vi "AutoDrive.vi"(10 "Target":dbl, 11 "Drive Effort":dbl) -> ()   [LabVIEW 2017]
uses:
  2017_Steamworks/Programming_Team/Competition/Worlds/Labview/Global 2.vi
  <vilib>/Rock Robotics/WPI/ThirdParty/Phoenix-LabVIEW/Motor Controller/Controls/CTRE_Phoenix_MotorControl_ControlMode.ctl
panel:
  in  "Scaling Factor":dbl
  in  "kD":dbl
  in  "kP":dbl
  in  "Scaling Factor":dbl=16.0 format="%#_13g"
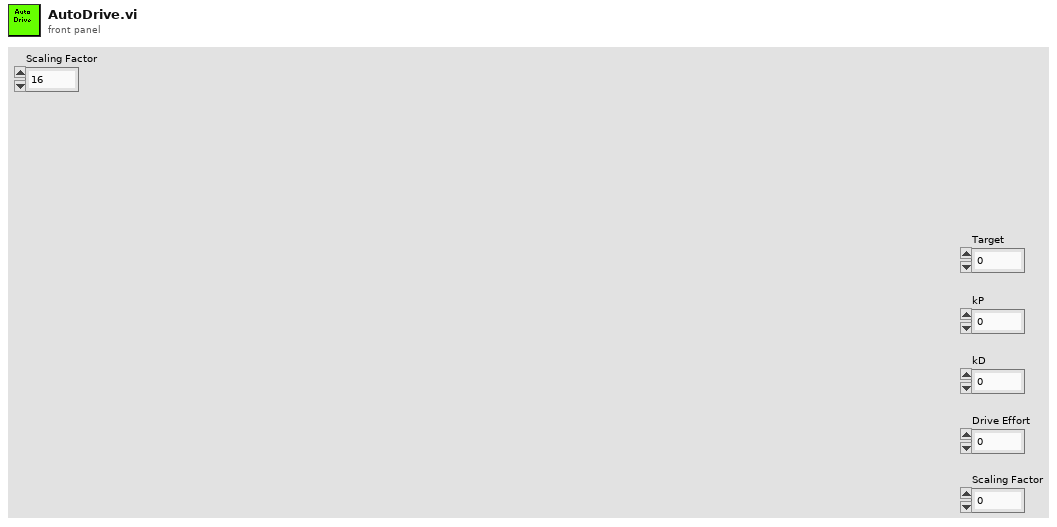
[diagram p1: front panel]
types:
  T1 = typedef "CTRE_Phoenix_MotorControl_ControlMode.ctl" = u16
  T2 = typedef "WPI_MotorControlDeviceRef.ctl" = cluster{"DeviceStatus":errorcluster, "Type":T3, "PWM":cluster{"PWM Channel":T4, "DeadBand":T5}, "CAN":cluster{"Device Number":u8, "SetOutput VI Ref":variant, "GetOutput VI Ref":variant, "Enable VI Ref":variant, "Disable VI Ref":variant, "Data":variant}, "Invert":bool, "DIO PWM":cluster{"PWM \"Enable\" Channel":T4, "DIOChannel":T6, "PWM Rate":dbl}}
  T3 = typedef "WPI_MotorControlType.ctl" = enum16{"PWM", "CAN", "DIO PWM"}
  T4 = typedef "FPGA_DIOPWMChannel.ctl" = enum8{"PWM 0", "PWM 1", "PWM 2", "PWM 3", "PWM 4", "PWM 5", "PWM 6", "PWM 7", "PWM 8", "PWM 9", "PWM MXP 0", "PWM MXP 1", "PWM MXP 2", "PWM MXP 3", "PWM MXP 4", "PWM MXP 5", "PWM MXP 6", "PWM MXP 7", "PWM MXP 8", "PWM MXP 9", "Invalid"}
  T5 = typedef "WPI_PWMDeadband.ctl" = cluster{"Name":string, "maxPositivePwm":i32, "minPositivePwm":i32, "centerPwm":i32, "maxNegativePwm":i32, "minNegativePwm":i32, "angularRange":u16}
  T6 = typedef "FPGA_DIOChannel.ctl" = enum8{"DIO 0", "DIO 1", "DIO 2", "DIO 3", "DIO 4", "DIO 5", "DIO 6", "DIO 7", "DIO 8", "DIO 9", "DIO MXP 0", "DIO MXP 1", "DIO MXP 2", "DIO MXP 3", "DIO MXP 4", "DIO MXP 5", "DIO MXP 6", "DIO MXP 7", "DIO MXP 8", "DIO MXP 9", "DIO MXP 10", "DIO MXP 11", "DIO MXP 12", "DIO MXP 13", "DIO MXP 14", "DIO MXP 15", "SPI Port CS1", "SPI Port CS2", "SPI Port CS3", "SPI Port MISO", "SPI Port MOSI", "Invalid"}
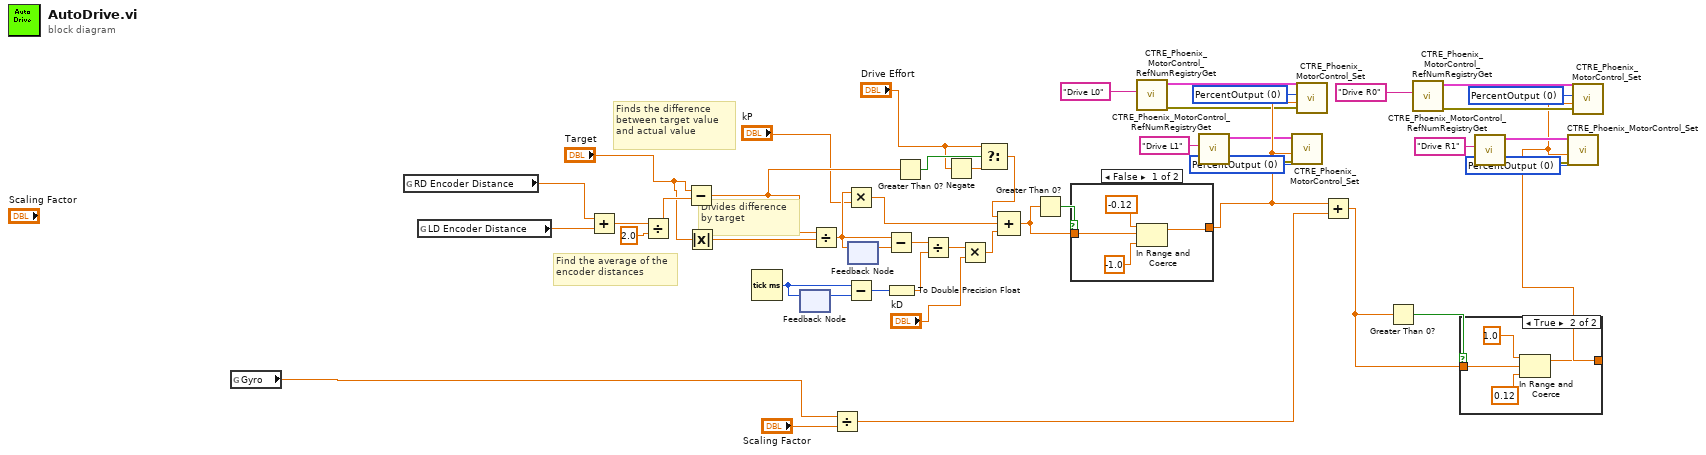
[diagram p0: block diagram]
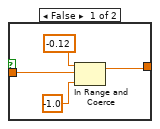
[diagram p2: hidden frame]
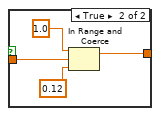
[diagram p3: hidden frame]
diagram:
  w1 = T1 0 items=["PercentOutput"=0, "Position"=1, "Velocity"=2, "Current"=3, "Follower"=5, "MotionProfile"=6, "MotionMagic"=7, "MotionMagicArc"=8, "MotionProfileArc"=10, "Disabled"=15] ("Control Mode")
  w2 = T1 0 items=["PercentOutput"=0, "Position"=1, "Velocity"=2, "Current"=3, "Follower"=5, "MotionProfile"=6, "MotionMagic"=7, "MotionMagicArc"=8, "MotionProfileArc"=10, "Disabled"=15] ("Control Mode")
  w3 = T1 0 items=["PercentOutput"=0, "Position"=1, "Velocity"=2, "Current"=3, "Follower"=5, "MotionProfile"=6, "MotionMagic"=7, "MotionMagicArc"=8, "MotionProfileArc"=10, "Disabled"=15] ("Control Mode")
  w4 = T1 0 items=["PercentOutput"=0, "Position"=1, "Velocity"=2, "Current"=3, "Follower"=5, "MotionProfile"=6, "MotionMagic"=7, "MotionMagicArc"=8, "MotionProfileArc"=10, "Disabled"=15] ("Control Mode")
  # "Divides difference by target"
  # "Finds the difference between target value and actual value"
  # "Find the average of the encoder distances"
  n1 = global read "Global 2.vi" "Gyro"() -> (w46:dbl)
  n2 = global read "Global 2.vi" "RD Encoder Distance"() -> (w30:dbl)
  n3 = global read "Global 2.vi" "LD Encoder Distance"() -> (w31:dbl)
  n4 = Add(x=w30, y=w31) -> (x+y=w45:dbl)
  n5 = Divide(x=w45, y=2.0) -> (x/y=w43:dbl)
  n6 = Subtract(x="Target", y=w43) -> (x-y=w25:dbl)
  n7 = Absolute Value(x="Target") -> (abs(x)=w27:dbl)
  n8 = Tick Count (ms)() -> (millisecond timer value=w40:u32)
  n9 = feedback #1() -> (w41:u32)  [unwired: 1 in]
  n10 = feedback-in #1(w40) -> ()
  n11 = Divide(x=w25, y=w27) -> (x/y=w26:dbl)
  n12 = Divide(x=w46, y="Scaling Factor") -> (x/y=w47:dbl)
  n13 = Multiply(x=w26, y="kP") -> (x*y=w35:dbl)
  n14 = Subtract(x=w40, y=w41) -> (x-y=w38:u32)
  n15 = feedback #2() -> (w42:dbl)  [unwired: 1 in]
  n16 = feedback-in #2(w26) -> ()
  n17 = Subtract(x=w26, y=w42) -> (x-y=w39:dbl)
  n18 = To Double Precision Float(number=w38) -> (double precision float=w37:dbl)
  n19 = Greater Than 0?(x=w25) -> (x > 0?=w24:bool)
  n20 = Divide(x=w39, y=w37) -> (x/y=w36:dbl)
  n21 = Negate(x="Drive Effort") -> (-x=w23:dbl)
  n22 = Multiply(x=w36, y="kD") -> (x*y=w34:dbl)
  n23 = Select(t="Drive Effort", s=w24, f=w23) -> (s? t:f=w22:dbl)
  n24 = Compound Arithmetic op=ADD(w22, w35, w34) -> (w32:dbl)
  n25 = Greater Than 0?(x=w32) -> (x > 0?=w33:bool)
  n26 = case shown="False" w33 {
    tunnel: [w50 w55] -> w17
    tunnel: w32 -> [w51 w54]
    frame False {
      n27 = In Range and Coerce(upper limit=-0.12, x=w51, lower limit=-1.0) -> (coerced(x)=w50:dbl)  [unwired: 1 out]
    }
    frame True {
      n28 = In Range and Coerce(upper limit=1.0, x=w54, lower limit=0.12) -> (coerced(x)=w55:dbl)  [unwired: 1 out]
    }
  }
  n29 = call <vilib>:"CTRE_Phoenix_MotorControl_RefNumRegistryGet.vi"("refnum name"="Drive L0") -> ("error out"=w12:errorcluster, "PhoenixMotorControlDevRef"=w13:T2)  [unwired: 9 in]
  n30 = call <vilib>:"CTRE_Phoenix_MotorControl_RefNumRegistryGet.vi"("refnum name"="Drive L1") -> ("error out"=w15:errorcluster, "PhoenixMotorControlDevRef"=w16:T2)  [unwired: 9 in]
  n31 = call <vilib>:"CTRE_Phoenix_MotorControl_Set.vi"("error in (no error)"=w15, "Output"=w17, "Control Mode"=w3, "PhoenixMotorControlDevRef"=w16) -> ()  [unwired: 6 in, 2 out]
  n32 = call <vilib>:"CTRE_Phoenix_MotorControl_Set.vi"("error in (no error)"=w12, "Output"=w17, "Control Mode"=w4, "PhoenixMotorControlDevRef"=w13) -> ()  [unwired: 6 in, 2 out]
  n33 = Add(x=w17, y=w47) -> (x+y=w28:dbl)
  n34 = Greater Than 0?(x=w28) -> (x > 0?=w29:bool)
  n35 = call <vilib>:"CTRE_Phoenix_MotorControl_RefNumRegistryGet.vi"("refnum name"="Drive R0") -> ("error out"=w6:errorcluster, "PhoenixMotorControlDevRef"=w7:T2)  [unwired: 9 in]
  n36 = case shown="True" w29 {
    tunnel: [w58 w63] -> w5
    tunnel: w28 -> [w59 w62]
    frame False {
      n37 = In Range and Coerce(upper limit=-0.12, x=w59, lower limit=-1.0) -> (coerced(x)=w58:dbl)  [unwired: 1 out]
    }
    frame True {
      n38 = In Range and Coerce(upper limit=1.0, x=w62, lower limit=0.12) -> (coerced(x)=w63:dbl)  [unwired: 1 out]
    }
  }
  n39 = call <vilib>:"CTRE_Phoenix_MotorControl_RefNumRegistryGet.vi"("refnum name"="Drive R1") -> ("error out"=w9:errorcluster, "PhoenixMotorControlDevRef"=w10:T2)  [unwired: 9 in]
  n40 = call <vilib>:"CTRE_Phoenix_MotorControl_Set.vi"("error in (no error)"=w9, "Output"=w5, "Control Mode"=w1, "PhoenixMotorControlDevRef"=w10) -> ()  [unwired: 6 in, 2 out]
  n41 = call <vilib>:"CTRE_Phoenix_MotorControl_Set.vi"("error in (no error)"=w6, "Output"=w5, "Control Mode"=w2, "PhoenixMotorControlDevRef"=w7) -> ()  [unwired: 6 in, 2 out]
